vi "target - multi rate - variables - fileIO.vi"   [LabVIEW 2021]
uses:
  <vilib>/Platform/TimedLoop/XDataNode/timing_clust.ctl
  <vilib>/Platform/TimedLoop/XDataNode/nitl_modes.ctl
  <vilib>/Platform/TimedLoop/XDataNode/wakeup.ctl
  <vilib>/Platform/TimedLoop/XDataNode/XDataNode.xnode
  <vilib>/Platform/TimedLoop/XDataNode/XDNodeRunTimeDep.lvlib
panel:
  # "The Network Variable Engine and Variable Client Support must be installed on the RT target\nfor this application to function properly. If the Network Variable Engine is not supported on\nthe target (e.g.  FP-2000 with <32MB of RAM), open the project and move the variable library\nto My Computer in the project. Doing this will deploy the variables to localhost but\nwill still require that Variable Client Support be installed on the RT target."
types:
  T1 = enum16{"open", "replace", "create", "open or create", "replace or create", "replace or create with confirmation"}
  T2 = typedef "XDNodeRunTimeDep.lvlib/timing_clust.ctl" = cluster{"Expected End [f-1]":u64, "Actual End [f-1]":u64, "Finished Late? [f-1]":bool, "Expected End [i-1]":u64, "Actual End [i-1]":u64, "Finished Late? [i-1]":bool, "Expected Start [i]":u64, "Actual Start [i]":u64, "Expected Start [f]":u64, "Actual Start [f]":u64, "Source Name":string, "Structure Name":string, "Period":i64, "Deadline":i64, "Offset":i64, "Start":i64, "Priority":i32, "Timeout":i32, "Mode":T3, "Wakeup Reason":T4, "Error":errorcluster, "Source Type":string, "Secondary Source Type":string, "Global End Time":u64, "Global Start Time":u64, "Frame Duration":u64, "Iteration Duration":u64, "Assigned CPU":i32, "I/O Scan Engine Mode":u32}
  T3 = typedef "XDNodeRunTimeDep.lvlib/nitl_modes.ctl" = enum32{"No Change", "Process missed periods, maintain original phase", "Discard missed periods, maintain original phase", "Process missed periods, ignore original phase", "Discard missed periods, ignore original phase"}
  T4 = typedef "XDNodeRunTimeDep.lvlib/wakeup.ctl" = enum32{"Normal", "Aborted", "Asynchronous wakeup", "Timing source error", "Timed loop error", "Timeout"}
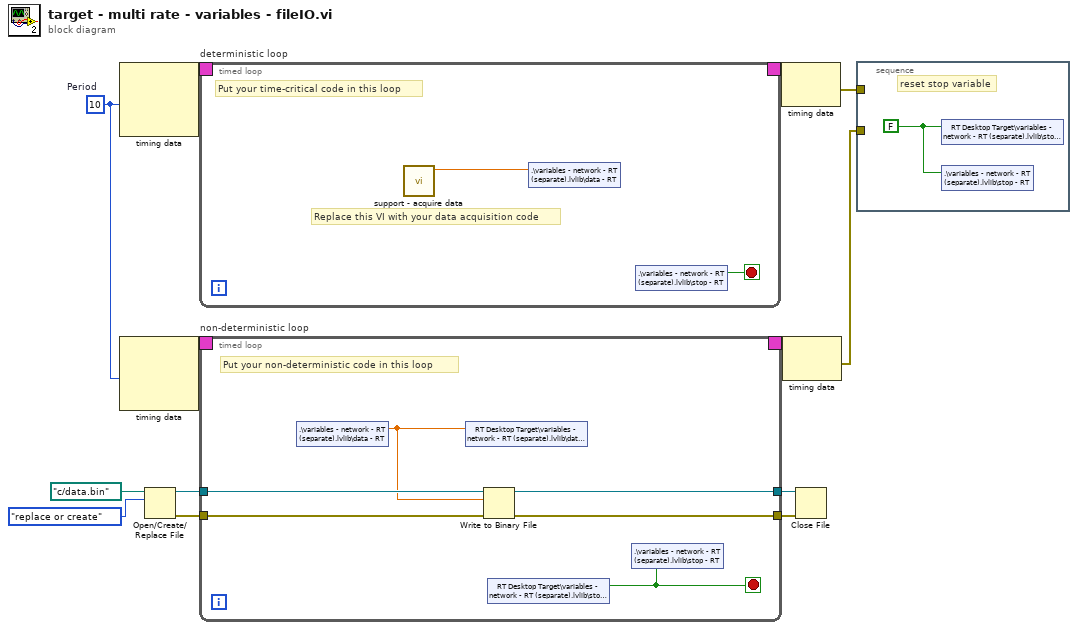
[diagram p0: block diagram]
diagram:
  w3 = i64 10  # Period
  n1 = node-c288 ("Input Node")(w3) -> (w13:T2)  [unwired: 2 in]
  n2 = node-c288 ("Input Node")(w3) -> (w11:T2)  [unwired: 2 in]
  n3 = Open/Create/Replace File(file path (use dialog)=path "c:/data.bin", operation (0:open)=T1."replace or create") -> (refnum out=w5:refnum<file>, error out=w4:errorcluster)  [unwired: 4 in, 1 out]
  n4 = timed-loop "deterministic loop" {
    timing: w13 -> [_]
    timing-out: [_] -> w12
    stop <- w14 stop-if-true
    # "Replace this VI with your data acquisition code"
    # "Put your time-critical code in this loop"
    n5 = call <resource>:"support - acquire data.vi"() -> ("sin(x)"=w15:dbl)  [unwired: 10 in, 1 out]
    n6 = shared-variable ".\\variables - network - RT (separate).lvlib\\data - RT"(w15) -> ()  [unwired: 1 in, 1 out]
    n7 = shared-variable ".\\variables - network - RT (separate).lvlib\\stop - RT"() -> (w14:bool)  [unwired: 1 in, 1 out]
  }
  n8 = timed-loop "non-deterministic loop" {
    timing: w11 -> [_]
    timing-out: [_] -> w10
    tunnel: [w23] -> w7
    tunnel: [w22] -> w6
    tunnel: w5 -> [w21]
    tunnel: w4 -> [w20]
    stop <- w18 stop-if-true
    # "Put your non-deterministic code in this loop"
    n9 = shared-variable ".\\variables - network - RT (separate).lvlib\\data - RT"() -> (w19:dbl)  [unwired: 1 in, 1 out]
    n10 = shared-variable "RT Desktop Target\\variables - network - RT (separate).lvlib\\data - network"(w19) -> ()  [unwired: 1 in, 1 out]
    n11 = Write to Binary File(file (use dialog)=w21, data=w19, error in=w20) -> (refnum out=w23:refnum<file>, error out=w22:errorcluster)  [unwired: 3 in, 1 out]
    n12 = shared-variable "RT Desktop Target\\variables - network - RT (separate).lvlib\\stop - network"() -> (w18:bool)  [unwired: 1 in, 1 out]
    n13 = shared-variable ".\\variables - network - RT (separate).lvlib\\stop - RT"(w18) -> ()  [unwired: 1 in, 1 out]
  }
  n14 = node-c288 ("Output Node")(w12) -> (w2:errorcluster)
  n15 = node-c288 ("Output Node")(w10) -> (w1:errorcluster)
  n16 = Close File(refnum=w7, error in=w6) -> ()  [unwired: 2 out]
  n17 = stacked-sequence {
    tunnel: w2 -> [_]
    tunnel: w1 -> [_]
    frame #0 {
      w26 = FALSE
      # "reset stop variable"
      n18 = shared-variable "RT Desktop Target\\variables - network - RT (separate).lvlib\\stop - network"(w26) -> ()  [unwired: 1 in, 1 out]
      n19 = shared-variable ".\\variables - network - RT (separate).lvlib\\stop - RT"(w26) -> ()  [unwired: 1 in, 1 out]
    }
  }
